vi "ROIAverage.vi"(0 "Hitachi Cal":sgl[][](array[numeric]) format="%.2f", 1 "ROI (PramImage Subset co-ords)":T1 {"Subset TPI offset" format="%.2f"; "#TPI pts" format="%.2f"; "TPI start" format="%.2f"}, 7 "midband att":dbl[](array[numeric]) format="%.2f", 11 "slope att":dbl[](array[numeric]) format="%.2f") -> (4 "av cal int":dbl format="%.2f", 6 "av cal mb":dbl format="%.2f", 8 "av att mb":dbl format="%.2f", 10 "av att slope":dbl format="%.2f", 15 "number of pts":dbl format="%.2f")   [LabVIEW 2022 SP3]
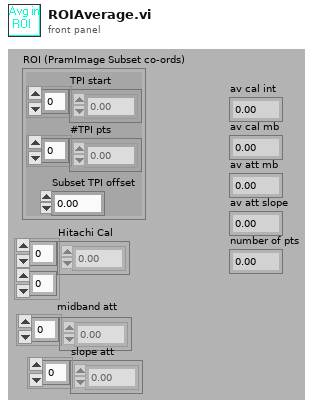
[diagram p1: front panel]
types:
  T1 = cluster{"TPI start":dbl[], "#TPI pts":dbl[], "Subset TPI offset":dbl}
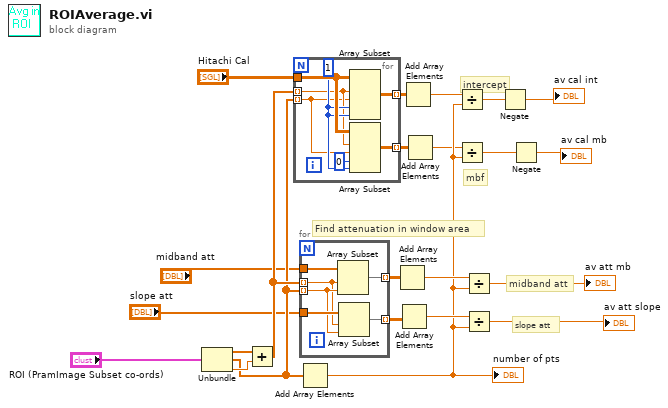
[diagram p0: block diagram]
diagram:
  # "mbf"
  # "intercept"
  # "slope att"
  # "midband att"
  # "Find attenuation in window area"
  n1 = Unbundle("ROI (PramImage Subset co-ords)") -> ("TPI start"=w20:dbl[], "#TPI pts"=w11:dbl[], "Subset TPI offset"=w21:dbl)
  n2 = Add(x=w20, y=w21) -> (x+y=w12:dbl[])
  n3 = for {
    tunnel: "Hitachi Cal" -> [w30]
    tunnel: [w27] -> w10 mode=indexing
    tunnel: [w26] -> w9 mode=indexing
    tunnel: w12 -> [w25] mode=indexing
    tunnel: w11 -> [w24] mode=indexing
    w29 = 1
    n4 = Array Subset(array=w30, index (row)=w25, length (row)=w24, index (col)=w29, length (col)=w29) -> (w27:sgl[][])
    n5 = Array Subset(array=w30, index (row)=w25, length (row)=w24, index (col)=0, length (col)=w29) -> (w26:sgl[][])
  }
  n6 = for {
    tunnel: "slope att" -> [w36]
    tunnel: "midband att" -> [w35]
    tunnel: w12 -> [w33] mode=indexing
    tunnel: w11 -> [w34] mode=indexing
    tunnel: [w32] -> w19 mode=indexing
    tunnel: [w31] -> w18 mode=indexing
    n7 = Array Subset(array=w35, index=w33, length=w34) -> (w32:dbl[])
    n8 = Array Subset(array=w36, index=w33, length=w34) -> (w31:dbl[])
  }
  n9 = Add Array Elements(numeric array=w11) -> (sum=w15:dbl)
  "number of pts" <- w15
  n10 = Add Array Elements(numeric array=w19) -> (sum=w17:dbl)
  n11 = Add Array Elements(numeric array=w18) -> (sum=w16:dbl)
  n12 = Add Array Elements(numeric array=w10) -> (sum=w8:sgl)
  n13 = Add Array Elements(numeric array=w9) -> (sum=w7:sgl)
  n14 = Divide(x=w8, y=w15) -> (x/y=w22:dbl)
  n15 = Divide(x=w7, y=w15) -> (x/y=w23:dbl)
  n16 = Divide(x=w17, y=w15) -> (x/y=→"av att mb":dbl)
  n17 = Divide(x=w16, y=w15) -> (x/y=→"av att slope":dbl)
  n18 = Negate(x=w22) -> (-x=→"av cal int":dbl)
  n19 = Negate(x=w23) -> (-x=→"av cal mb":dbl)
